vi "Get Slave Device Info.vi"(0 "System no.":i32=1, 5 "error in":errorcluster) -> (14 "Slave Device Info":cluster{"Slave ID":i32, "*IDN? Answer":string}[](array[cluster]), 19 "error out":errorcluster)   [LabVIEW 2020]
doc: "This VI queries VER? and lists all connected DaisyChain slave devices."
uses:
  <vilib>/regexp/Match Regular Expression.xnode
panel:
  # "This VI queries VER? and lists all connected DaisyChain slave devices."
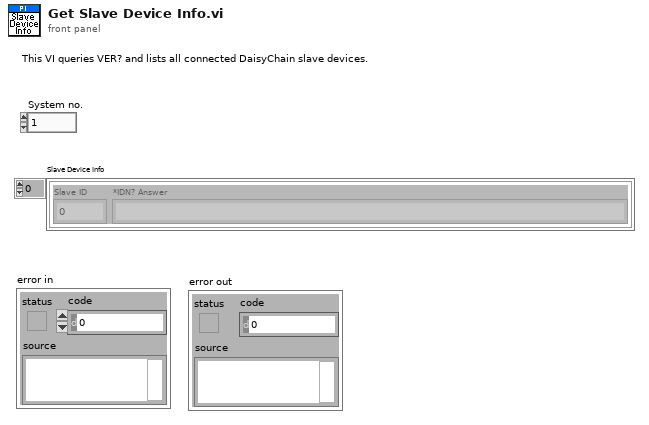
[diagram p1: front panel]
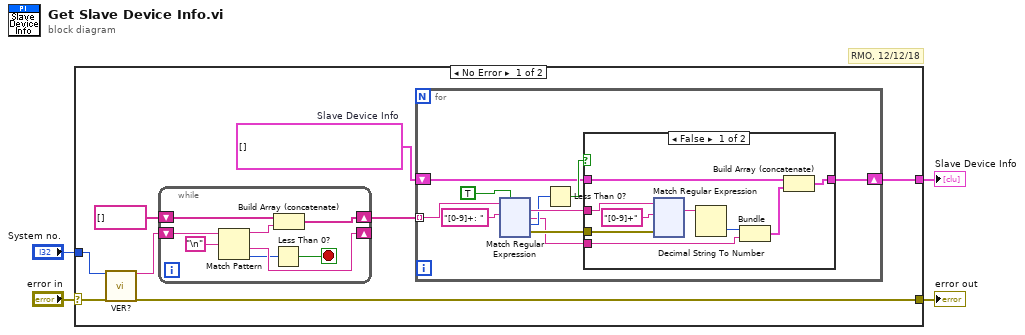
[diagram p0: block diagram]
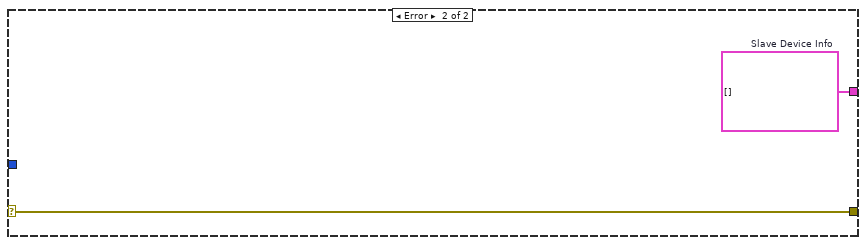
[diagram p3: hidden frame]
diagram:
  # "RMO, 12/12/18"
  n1 = case shown="No Error" "error in" {
    selector: "error in" -> [w5 w270]
    tunnel: [w12 w269] -> w4
    tunnel: [w8 w270] -> w3
    tunnel: "System no." -> [w6 _]
    frame No Error {
      w11 = cluster{"Slave ID":i32, "*IDN? Answer":string}[] []  # Slave Device Info
      n2 = call "VER?.vi"("System no."=w6, "error in"=w5) -> ("Firmware version"=w10:string, "error out"=w8:errorcluster)  [unwired: 16 out]
      n3 = while {
        shift-right: [w264] -> _
        shift-left: w10 -> [w268]
        shift-right: [w263] -> w9
        shift-left: string[] [] -> [w266]
        stop <- w261 stop-if-true
        n4 = Match Pattern(string=w268, regular expression="\n") -> (before substring=w265:string, after substring=w264:string, offset past match=w262:i32)  [unwired: 2 out]
        n5 = Less Than 0?(x=w262) -> (x < 0?=w261:bool)
        n6 = Build Array (concatenate)(w266, w265) -> (w263:string[])
      }
      n7 = for {
        tunnel: w9 -> [w22] mode=indexing
        shift-right: [w13] -> w12
        shift-left: w11 -> [w14]
        n8 = xnode "Match Regular Expression"("input string"=w22, "regular expression"="[0-9]+: ", "ignore case? (F)"=TRUE) -> ("whole match"=w18:string, "after match"=w15:string, "offset past match"=w17:i32, "error out"=w19:errorcluster)  [unwired: 2 in, 2 out]
        n9 = Less Than 0?(x=w17) -> (x < 0?=w16:bool)
        n10 = case shown="False" w16 {
          tunnel: w19 -> [w31 _]
          tunnel: w18 -> [w30 _]
          tunnel: w15 -> [w26 _]
          tunnel: w14 -> [w24 w146]
          tunnel: [w23 w146] -> w13
          frame False {
            n11 = xnode "Match Regular Expression"("input string"=w30, "regular expression"="[0-9]+", "error in"=w31) -> ("whole match"=w28:string)  [unwired: 1 in, 6 out]
            n12 = Decimal String To Number(string=w28) -> (number=w27:i32)  [unwired: 3 out]
            n13 = Bundle(w27, "after match"=w26) -> (w25:cluster{i32, "after match":string})  [unwired: 1 out]
            n14 = Build Array (concatenate)(w24, w25) -> (w23:cluster{"Slave ID":i32, "after match":string}[])
          }
          frame True {
          }
        }
      }
    }
    frame Error {
      w269 = cluster{"Slave ID":i32, "*IDN? Answer":string}[] []  # Slave Device Info
    }
  }
  "Slave Device Info" <- w4
  "error out" <- w3
